vi "Tool Stroker Osctun decoder.vi"(0 "Force NA(F)":bool, 7 "Valv Relay code":u8 format="%.0b") -> (4 "Ongoing":T1, 6 "Ending":T1)   [LabVIEW 2011]
uses:
  Measurments Handling/Status Digitalish.ctl
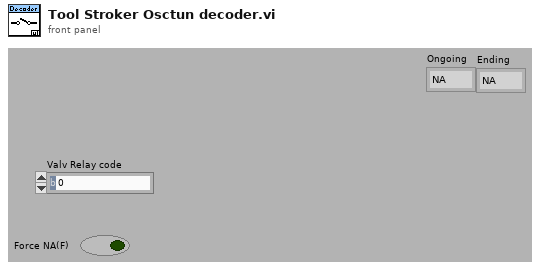
[diagram p1: front panel]
types:
  T1 = typedef "Status Digitalish.ctl" = enum16{"NA", "False", "True"}
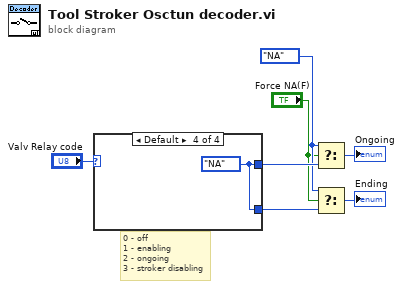
[diagram p0: block diagram]
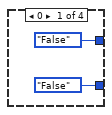
[diagram p2: hidden frame]
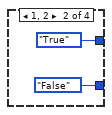
[diagram p3: hidden frame]
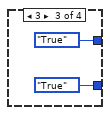
[diagram p4: hidden frame]
diagram:
  w5 = Status_Digitalish."NA" ("t")
  # "0 - off\n1 - enabling\n2 - ongoing\n3 - stroker disabling"
  n1 = case shown="Default" "Valv Relay code" {
    tunnel: [Status_Digitalish."False" ("Status") Status_Digitalish."True" ("Status") Status_Digitalish."True" ("Status") w14] -> w6
    tunnel: [Status_Digitalish."False" ("Status") Status_Digitalish."False" ("Status") Status_Digitalish."True" ("Status") w14] -> w3
    frame 0 {
    }
    frame 1, 2 {
    }
    frame 3 {
    }
    frame Default {
      w14 = Status_Digitalish."NA" ("Status")
    }
  }
  n2 = Select(t=w5, s="Force NA(F)", f=w6) -> (s? t:f=→"Ongoing":T1)
  n3 = Select(t=w5, s="Force NA(F)", f=w3) -> (s? t:f=→"Ending":T1)
